vi "Create.vi"(8 "error in":errorcluster, 11 "Type Definition":refnum<class "Type Definition.lvclass">) -> (0 "error out":errorcluster, 3 "PV Data":refnum<class "PV Data.lvclass">)   [LabVIEW 2020, in "PV Access.lvlib" / "PV Data.lvlib" / "PV Data.lvclass"]
uses:
  PV Data.lvclass
  Type Definition/Type Definition.lvclass
  PV Access.lvlib
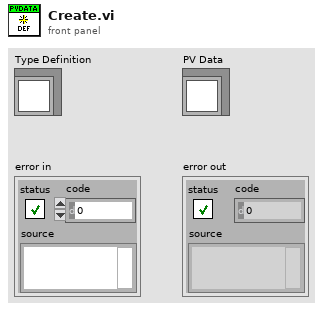
[diagram p1: front panel]
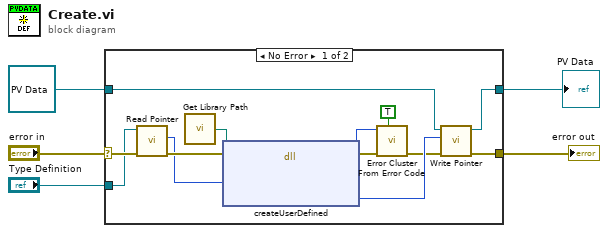
[diagram p0: block diagram]
diagram:
  n1 = case shown="No Error" "error in" {
    selector: "error in" -> [w9 w20]
    tunnel: [w11 w20] -> w5
    tunnel: refnum<class "PV Data.lvclass"> refnum ("PV Data in") -> [w13 w19]
    tunnel: [w12 w19] -> w2
    tunnel: "Type Definition" -> [w7 _]
    frame No Error {
      n2 = call-dynamic "Read Pointer.vi"("error in (no error)"=w9, "Pointer Base in"=w7) -> ("error out"=w8:errorcluster, "Pointer"=w6:i64)  [unwired: 7 in, 1 out]
      n3 = call "Get Library Path.vi"() -> ("Path"=w15:path)  [unwired: 1 in]
      n4 = dll-call lib="?" fn="createUserDefined" ("createNT Scalar")(path in=w15, error in=w8, "type def"=w6) -> (error out=w17:errorcluster, "err_code"=w16:i32, "value"=w14:i64)  [unwired: 3 in, 1 out]
      n5 = call <vilib>:"Error Cluster From Error Code.vi"("show call chain? (False)"=TRUE, "error in (no error)"=w17, "error code (0)"=w16) -> ("error out"=w10:errorcluster)  [unwired: 6 in]
      n6 = call-dynamic "Write Pointer.vi"("error in (no error)"=w10, "Pointer"=w14, "Pointer Base in"=w13) -> ("error out"=w11:errorcluster, "Pointer Base out"=w12:refnum<class "PV Data.lvclass">)  [unwired: 7 in]
    }
    frame Error {
    }
  }
  "error out" <- w5
  "PV Data" <- w2
